vi "SNMP Type Num to Type String.vi"(1 "Type":u8) -> (0 "StringForType":string)   [LabVIEW 2017]
doc: "This VI converts the numeric value for the SNMP data type to an ASCII string. For example, a value of 2 would be converted to INTEGER."
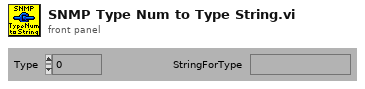
[diagram p1: front panel]
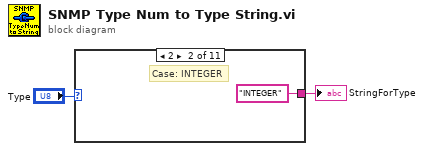
[diagram p0: block diagram]
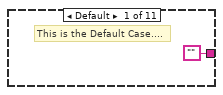
[diagram p2: hidden frame]
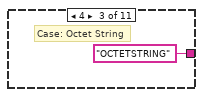
[diagram p3: hidden frame]
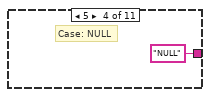
[diagram p4: hidden frame]
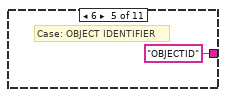
[diagram p5: hidden frame]
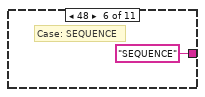
[diagram p6: hidden frame]
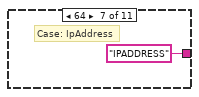
[diagram p7: hidden frame]
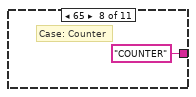
[diagram p8: hidden frame]
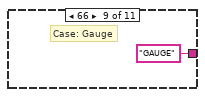
[diagram p9: hidden frame]
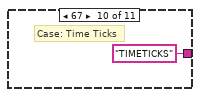
[diagram p10: hidden frame]
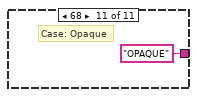
[diagram p11: hidden frame]
diagram:
  n1 = case shown="2" "Type" {
    tunnel: ["" "INTEGER" "OCTETSTRING" "NULL" "OBJECTID" "SEQUENCE" "IPADDRESS" "COUNTER" "GAUGE" "TIMETICKS" "OPAQUE"] -> w1
    frame Default {
      # "This is the Default Case...."
    }
    frame 2 {
      # "Case: INTEGER"
    }
    frame 4 {
      # "Case: Octet String"
    }
    frame 5 {
      # "Case: NULL"
    }
    frame 6 {
      # "Case: OBJECT IDENTIFIER"
    }
    frame 48 {
      # "Case: SEQUENCE"
    }
    frame 64 {
      # "Case: IpAddress"
    }
    frame 65 {
      # "Case: Counter"
    }
    frame 66 {
      # "Case: Gauge"
    }
    frame 67 {
      # "Case: Time Ticks"
    }
    frame 68 {
      # "Case: Opaque"
    }
  }
  "StringForType" <- w1
